vi "启动.vi"() -> ()   [LabVIEW 2016]
uses:
  <vilib>/NI/Progress Bar/Controls/Update Bar Actions.ctl
  <vilib>/NI/Progress Bar/Controls/Progress Bar Properties.ctl
  <vilib>/NI/Progress Bar/Progress Bar.lvlib
  API/update/update.lvlib
panel:
  out "exists?":bool
  out "error out":errorcluster
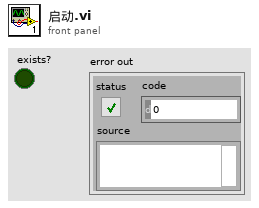
[diagram p1: front panel]
types:
  T1 = enum32{"Invalid", "Standard", "Closed", "Hidden", "Minimized", "Maximized"}
  T2 = typedef "Progress Bar.lvlib/Progress Bar Properties.ctl" = cluster{"Background Color":u32, "Installer Title":string, "Title Color":u32, "Action Text":string, "Text Color":u32, "Slider Value":u8, "Bar Color":u32, "Timeout":i32}
  T3 = typedef "Progress Bar.lvlib/Update Bar Actions.ctl" = enum16{"Add To Existing", "Set to Value"}
  T4 = cluster{"名称或相对路径":string, "MD5 message-digest":string}[]
  T5 = cluster{"host":string, "port":u16, "user":string, "password":string, "远端地址":string}
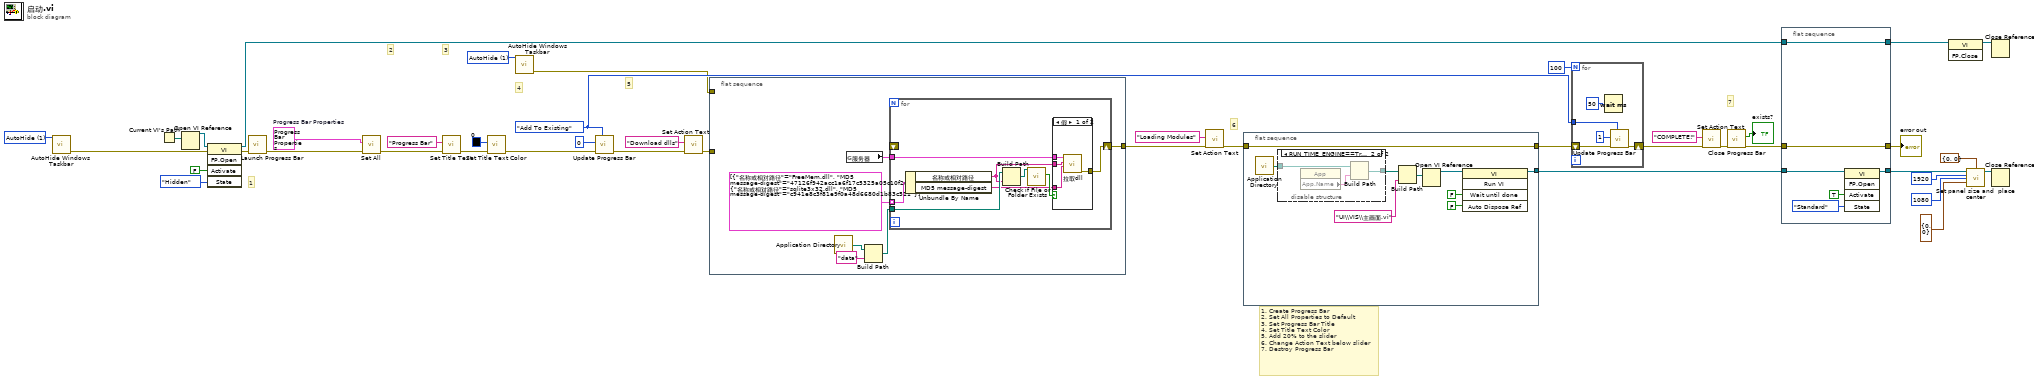
[diagram p0: block diagram]
diagram:
  w1 = u8 1 items=["AutoHide"=1, "AlwaysOnTop"=2] ("Operation")
  w10 = u8 1 items=["AutoHide"=1, "AlwaysOnTop"=2] ("Operation")
  w30 = T2 {"Background Color"=3381759, "Installer Title"="Progress", "Title Color"=0, "Action Text"="", "Text Color"=0, "Slider Value"=0, "Bar Color"=6618880, "Timeout"=10000}  # Progress Bar Properties
  w29 = Update_Bar_Actions."Add To Existing" ("Action")
  # "7"
  # "6"
  # "5"
  # "4"
  # "3"
  # "2"
  # "1"
  # "1. Create Progress Bar\n2. Set All Properties to Default\n3. Set Progress Bar Title\n4. Set Title Text Color\n5. Add 20% to the slider\n6. Change Action Text below slider\n7. Destroy Progress Bar"
  n1 = call "AutoHide Windows Taskbar.vi"("Operation"=w1) -> ("error out"=w2:errorcluster)  [unwired: 6 in]
  n2 = Current VI's Path() -> (path=w23:path)
  n3 = Open VI Reference(vi path=w23) -> (vi reference=w24:refnum<vi>)  [unwired: 5 in, 1 out]
  n4 = invoke class="VI" method="FP.Open"(reference=w24, error in=w2, "Activate"=FALSE ("激活？"), "State"=T1."Hidden" ("状态")) -> (reference out=w19:refnum<vi>, error out=w20:errorcluster)  [unwired: 1 in, 3 out]
  n5 = call <vilib>:"Launch Progress Bar.vi"("error in (no error)"=w20) -> ("error out"=w31:errorcluster)  [unwired: 9 in, 1 out]
  n6 = call <vilib>:"Set All.vi"("error in (no error)"=w31, "Progress Bar Properties (Default)"=w30) -> ("error out"=w38:errorcluster)  [unwired: 9 in]
  n7 = call <vilib>:"Set Title Text.vi"("error in (no error)"=w38, "Installer Title"="Progress Bar") -> ("error out"=w41:errorcluster)  [unwired: 9 in]
  n8 = call <vilib>:"Set Title Text Color.vi"("error in (no error)"=w41, "Color Box"=u32 0) -> ("error out"=w37:errorcluster)  [unwired: 9 in]
  n9 = call "AutoHide Windows Taskbar.vi"("Operation"=w10) -> ("error out"=w9:errorcluster)  [unwired: 6 in]
  n10 = call <vilib>:"Update Progress Bar.vi"("Action"=w29, "error in (no error)"=w37, "Value"=u8 0) -> ("error out"=w18:errorcluster)  [unwired: 8 in]
  n11 = call <vilib>:"Set Action Text.vi"("error in (no error)"=w18, "Action Text"="Download dlls") -> ("error out"=w16:errorcluster)  [unwired: 9 in]
  n12 = flat-sequence {
    tunnel: w16 -> [_]
    tunnel: [w43] -> w15
    tunnel: w9 -> [_]
    frame #0 {
      n13 = call <vilib>:"Application Directory.vi"() -> ("Application Directory"=w47:path)
      n14 = global read "系统设置全局变量.vi" "服务器"() -> (w44:T5)
      n15 = Build Path(base path=w47, name or relative path="data" ("名称或相对路径")) -> (appended path=w45:path)
      n16 = for {
        tunnel: T4 [{"名称或相对路径"="FreeMem.dll", "MD5 message-digest"="47126f942acc1a6f17c5325a05c10f2e"}, {"名称或相对路径"="sqlite3x32.dll", "MD5 message-digest"="c941e8c3f81e9f0a48d6680d1b83c511"}] -> [w55] mode=indexing
        tunnel: w45 -> [w54]
        tunnel: w44 -> [w53]
        shift-right: [w49] -> w43
        shift-left: _ -> [_]
        n17 = Unbundle By Name(w55) -> ("名称或相对路径"=w51:string, "MD5 message-digest"=w50:string)
        n18 = Build Path(base path=w54, name or relative path=w51) -> (appended path=w56:path)
        n19 = call <vilib>:"Check if File or Folder Exists.vi"("path"=w56) -> ("file or folder exists?"=w52:bool)  [unwired: 8 in, 2 out]
        n20 = case shown="假" w52 {
          tunnel: w53 -> [w60 _]
          tunnel: w51 -> [w59 _]
          tunnel: w50 -> [w58 _]
          tunnel: [w57 _] -> w49
          frame False {
            n21 = call "拉取dll.vi"("MD5 message-digest"=w58, "名称或相对路径"=w59, "服务器"=w60) -> ("error out"=w57:errorcluster)  [unwired: 8 in]
          }
          frame True {
          }
        }
      }
    }
  }
  n22 = call <vilib>:"Set Action Text.vi"("error in (no error)"=w15, "Action Text"="Loading Modules") -> ("error out"=w36:errorcluster)  [unwired: 9 in]
  n23 = flat-sequence {
    tunnel: w36 -> [w69]
    tunnel: [w69] -> w34
    tunnel: [w63] -> w14
    frame #0 {
      n24 = call <vilib>:"Application Directory.vi"() -> ("Application Directory"=w68:path)
      n25 = disable-structure shown="RUN_TIME_ENGINE==True" {
        disable-tunnel: w68 -> [w70 w73]
        disable-tunnel: [w70 w71] -> w66
        frame condition #0 (active) {
        }
        frame condition #1 {
          n26 = property class="App"() -> ("App.Name"=w72:string)  [unwired: 2 in, 2 out]
          n27 = Build Path(base path=w73, name or relative path=w72) -> (appended path=w71:path)
        }
      }
      n28 = Build Path(base path=w66, name or relative path="UI\\VIS\\主画面.vi" ("名称或相对路径")) -> (appended path=w62:path)
      n29 = Open VI Reference(vi path=w62) -> (vi reference=w61:refnum<vi>)  [unwired: 5 in, 1 out]
      n30 = invoke class="VI" method="Run VI"(reference=w61, "Wait until done"=FALSE ("结束前等待"), "Auto Dispose Ref"=FALSE ("自动销毁引用")) -> (reference out=w63:refnum<vi>)  [unwired: 2 in, 4 out]
    }
  }
  n31 = for {
    N: 100 ("Value") -> [_]
    tunnel: w29 -> [w75]
    shift-right: [w78] -> w33
    shift-left: w34 -> [w77]
    n32 = Wait (ms)(milliseconds to wait=u32 50) -> ()  [unwired: 1 out]
    n33 = call <vilib>:"Update Progress Bar.vi"("Action"=w75, "error in (no error)"=w77, "Value"=u8 1) -> ("error out"=w78:errorcluster)  [unwired: 8 in]
  }
  n34 = call <vilib>:"Set Action Text.vi"("error in (no error)"=w33, "Action Text"="COMPLETE!") -> ("error out"=w13:errorcluster)  [unwired: 9 in]
  n35 = call <vilib>:"Close Progress Bar.vi"("error in (no error)"=w13) -> ("error out"=w12:errorcluster, "exists?"=→"exists?":bool)  [unwired: 9 in]
  n36 = flat-sequence {
    tunnel: w12 -> [w84]
    tunnel: [w84] -> w11
    tunnel: [w83] -> w25
    tunnel: w19 -> [w83]
    tunnel: w14 -> [w82]
    tunnel: [w81] -> w4
    frame #0 {
      n37 = invoke class="VI" method="FP.Open"(reference=w82, "Activate"=TRUE ("激活？"), "State"=T1."Standard" ("状态")) -> (reference out=w81:refnum<vi>)  [unwired: 2 in, 4 out]
    }
  }
  n38 = invoke class="VI" method="FP.Close"(reference=w25) -> (reference out=w26:refnum<vi>)  [unwired: 2 in, 2 out]
  n39 = call "Set panel size and  place center.vi"("VI引用句柄"=w4, "FP.WinOrigin in(H & V)"=cluster{"Horizontal":i16, "Vertical":i16} {"Horizontal"=0, "Vertical"=0}, "Panel Width"=1920, "Panel Height"=1080, "FP.Origin in(H & V)"=cluster{"Horizontal":i16, "Vertical":i16} {"Horizontal"=0, "Vertical"=0}) -> ("Application or VI Refnum"=w3:refnum<vi>)  [unwired: 9 in, 1 out]
  n40 = Close Reference(reference=w26) -> ()  [unwired: 1 in, 1 out]
  n41 = Close Reference(reference=w3) -> ()  [unwired: 1 in, 1 out]
  "error out" <- w11
